vi "Clear-object.vi"(8 "error in":errorcluster, 11 "UI ref.":refnum<data-value>) -> (0 "error IO":errorcluster)   [LabVIEW 2013, in "CameraVision.lvlib" / "CV-UI.lvclass"]
doc: "This function deletes the data from the various GUI graphs and displays. This avoids interference with data from a previous acquisition."
uses:
  CV-UI.lvclass
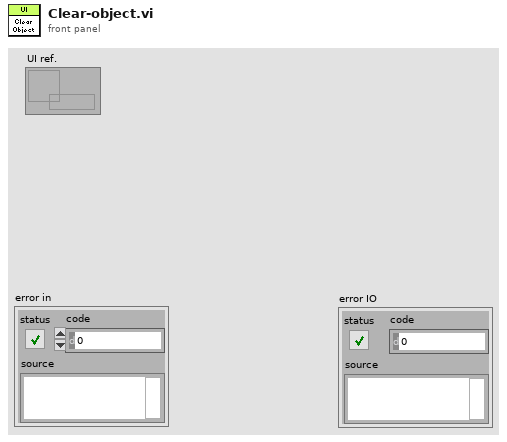
[diagram p1: front panel]
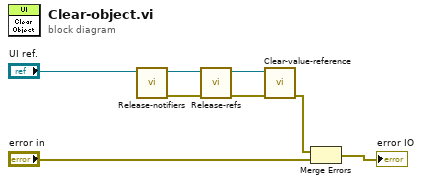
[diagram p0: block diagram]
diagram:
  n1 = call "Release-notifiers.vi"("UI ref. in"="UI ref.") -> ("error out"=w7:errorcluster, "UI ref."=w4:refnum<data-value>)  [unwired: 9 in]
  n2 = call "Release-refs.vi"("error in (no error)"=w7, "UI ref. in"=w4) -> ("error out"=w6:errorcluster, "UI ref."=w5:refnum<data-value>)  [unwired: 8 in]
  n3 = call "Clear-value-reference.vi"("error in (no error)"=w6, "UI ref."=w5) -> ("error out"=w3:errorcluster)  [unwired: 8 in, 1 out]
  n4 = Merge Errors(w3, "error in") -> (→"error IO":errorcluster)
